vi "Get Cluster Label Number.vi"(8 "error in":errorcluster, 11 "Ref in":refnum<vi>) -> (0 "error out":errorcluster, 2 "Label.Text":string)   [LabVIEW 2020, in "FakedArray.lvclass"]
uses:
  FakedArray.lvclass
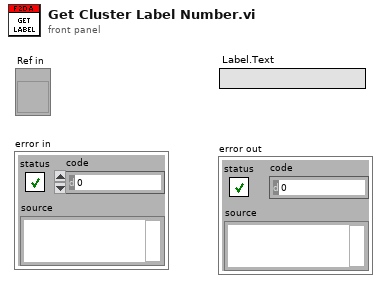
[diagram p1: front panel]
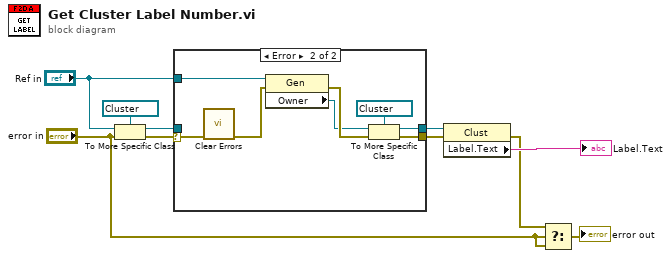
[diagram p0: block diagram]
diagram:
  n1 = To More Specific Class(target class=refnum<vi> refnum ("Clust Refnum"), reference="Ref in", error in="error in") -> (specific class reference=w6:refnum<vi>, error out=w8:errorcluster)
  n2 = case shown="Error" w8 {
    selector: w8 -> [w11 w19]
    tunnel: "Ref in" -> [_ w20]
    tunnel: w6 -> [w12 _]
    tunnel: [w12 w16] -> w5
    tunnel: [w11 w15] -> w4
    frame No Error {
    }
    frame Error {
      n3 = call <vilib>:"Clear Errors.vi"("error in (no error)"=w19) -> ("error out"=w14:errorcluster)  [unwired: 1 in, 5 out]
      n4 = property class="Gen"(reference=w20, error in=w14) -> (error out=w17:errorcluster, "Owner"=w13:refnum<vi>)  [unwired: 1 out]
      n5 = To More Specific Class(target class=refnum<vi> refnum ("Clust Refnum"), reference=w13, error in=w17) -> (specific class reference=w16:refnum<vi>, error out=w15:errorcluster)
    }
  }
  n6 = property class="Clust"(reference=w5, error in=w4) -> (error out=w2:errorcluster, "Label.Text"=→"Label.Text":string)  [unwired: 1 out]
  n7 = Select(t=w2, s="error in", f="error in") -> (s? t:f=→"error out":errorcluster)
